vi "Monitor-temperatura.vi"() -> ()   [LabVIEW 2018]
panel:
  in  "Temp Scale":bool
  out "TEMP Historical":dbl(graph)
  in  "POWER":bool
  # "ON"
  # "OFF"
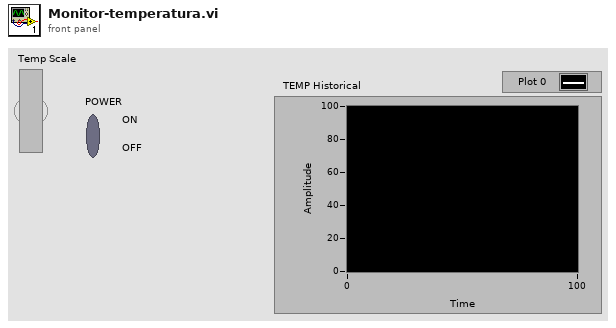
[diagram p1: front panel]
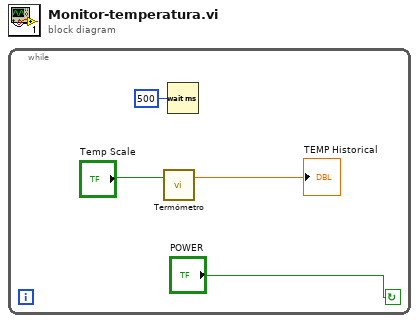
[diagram p0: block diagram]
diagram:
  n1 = while {
    stop <- "POWER" continue-if-true
    n2 = call "Termómetro.vi"("Temp Scale"="Temp Scale") -> ("Thermometer"=→"TEMP Historical":dbl)  [unwired: 2 in]
    n3 = Wait (ms)(milliseconds to wait=u32 500) -> ()  [unwired: 1 out]
  }
